vi "Set PanelVIRefs.vi"(8 "error in (no error)":errorcluster caption="错误输入（无错误）", 11 "PanelExample 输入":refnum<class "PanelExample.lvclass"> caption="DNL_LabVIEW Object in") -> (0 "error out":errorcluster caption="错误输出", 1 "VerticalPanel":refnum<vi>, 2 "HorizontalPanel":refnum<vi>, 3 "PanelExample 输出":refnum<class "PanelExample.lvclass"> caption="DNL_LabVIEW Object out")   [LabVIEW 2013, in "PanelExample.lvclass"]
uses:
  PanelExample.lvclass
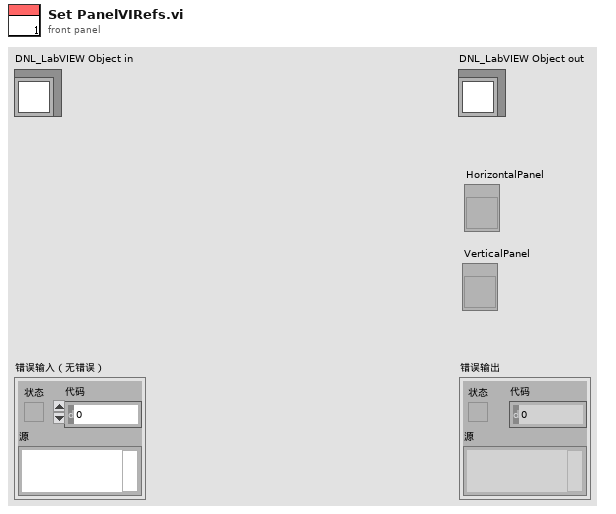
[diagram p1: front panel]
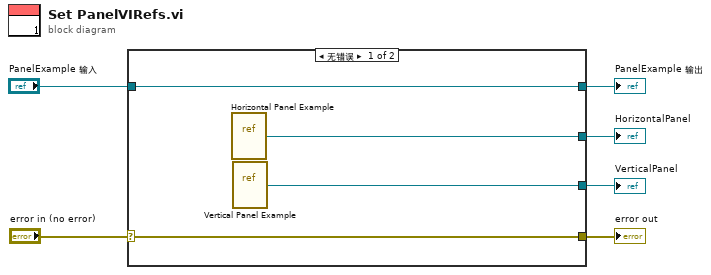
[diagram p0: block diagram]
diagram:
  n1 = case shown="无错误" "error in (no error)" {
    selector: "error in (no error)" -> [w8 w11]
    tunnel: [w10 _] -> w6
    tunnel: [w9 _] -> w5
    tunnel: [w8 w11] -> w3
    tunnel: "PanelExample 输入" -> [w7 w12]
    tunnel: [w7 w12] -> w1
    frame No Error {
      n2 = vi-ref "Horizontal Panel Example.vi"() -> (w9:refnum<vi>)
      n3 = vi-ref "Vertical Panel Example.vi"() -> (w10:refnum<vi>)
    }
    frame Error {
    }
  }
  "error out" <- w3
  "PanelExample 输出" <- w1
  "HorizontalPanel" <- w5
  "VerticalPanel" <- w6
